vi "Chessy_Drive_Main.vi"(0 "Speed_Main":dbl, 1 "Turning_Main":dbl, 5 "Speed_Limit":dbl, 7 "Turning_Limit":dbl, 12 "Quick_Turn":bool) -> (3 "Left_Motor":dbl format="%.2f", 14 "Right_Motor":dbl format="%.2f")   [LabVIEW 2014]
uses:
  General_VI/Global Var.vi
panel:
  out "Yaw 2":dbl(graph)
  in  "Tune_PID":bool
  out "Yaw":dbl(graph)
  in  "PID Turnin Gains":T1={"proportional gain (Kc)"=0.02, "integral time (Ti, min)"=0.0, "derivative time (Td, min)"=0.003} {"derivative time (Td, min)" format="%.3f"; "integral time (Ti, min)" format="%.3f"; "proportional gain (Kc)" format="%.3f"}
  out "XY Turning":cluster{"Turning X ":dbl[], "Turning Y":dbl[]}(graph)
  out "XY Speed":cluster{"Speed X":dbl[], "Speed Y":dbl[]}(graph)
  in  "Turning Scale":dbl=1.5
  in  "Turning Y":dbl[](array[numeric])=[-0.5, -0.3, -0.1, 0.0, 0.0, 0.0, 0.1, 0.3, 0.5]
  in  "Turning X":dbl[](array[numeric])=[-1.0, -0.75, -0.12, -0.1, 0.0, 0.1, 0.12, 0.75, 1.0]
  in  "Speed Y":dbl[](array[numeric])=[-0.6, -0.4, -0.15, 0.0, 0.0, 0.0, 0.15, 0.4, 0.6]
  in  "Speed X":dbl[](array[numeric])=[-1.0, -0.75, -0.06, -0.05, 0.0, 0.05, 0.06, 0.75, 1.0]
  in  "Turning_Hyd_Deadband":dbl=0.75
  in  "Speed_Hyd_Deadband":dbl=0.75
  out "Delta":dbl format="%.2f"
  # "Chessy Drive"
  # "This subystem takes turning and speed controls from a xbox joystick \nand creats left and right motor values"
  # "Tunning"
  # "Inputs"
  # "Test Points"
  # "Ouputs"
  # "Joystick Map (Lookup Table)"
  # "Hyp Cmd Deadband"
  # "Turning Power Mode"
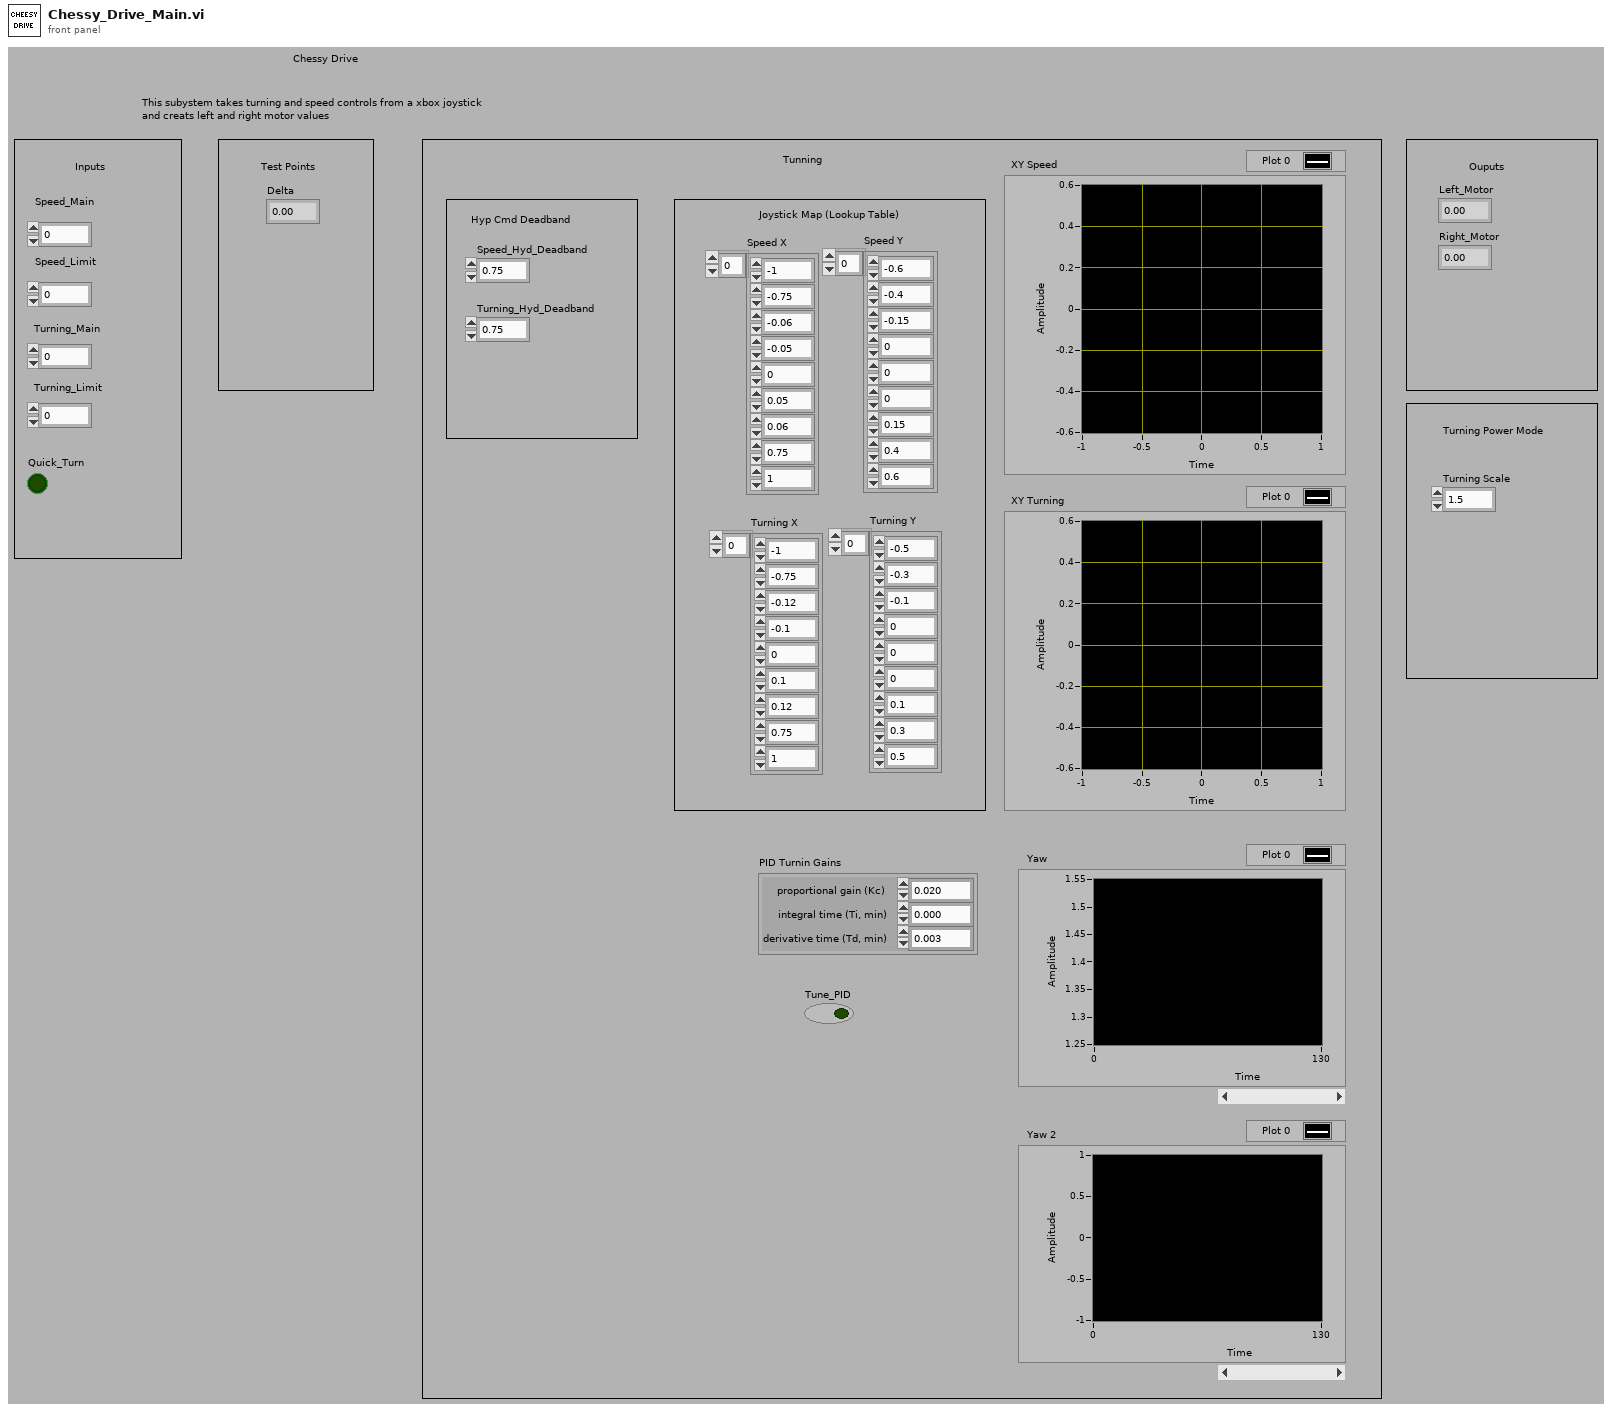
[diagram p1: front panel]
types:
  T1 = cluster{"proportional gain (Kc)":dbl, "integral time (Ti, min)":dbl, "derivative time (Td, min)":dbl}
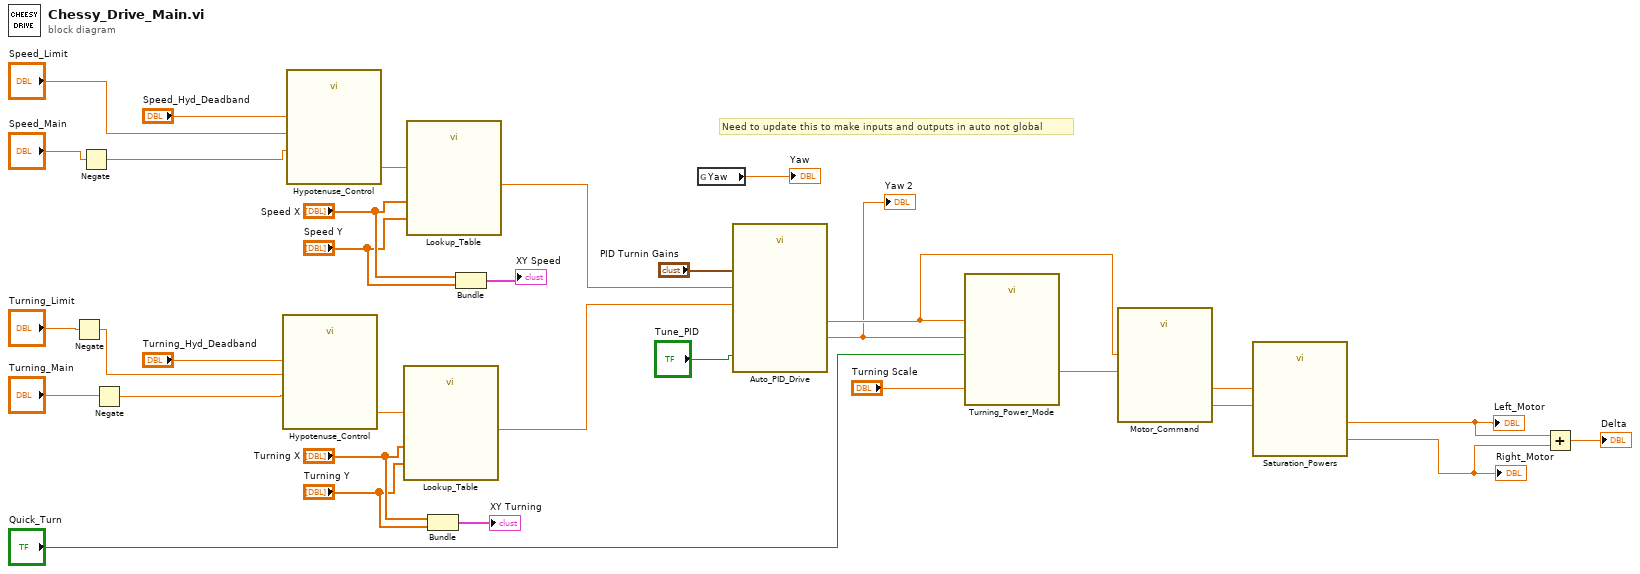
[diagram p0: block diagram]
diagram:
  # "Need to update this to make inputs and outputs in auto not global"
  n1 = Negate(x="Turning_Limit") -> (-x=w16:dbl)
  n2 = Negate(x="Speed_Main") -> (-x=w8:dbl)
  n3 = Negate(x="Turning_Main") -> (-x=w18:dbl)
  n4 = call "Hypotenuse_Control.vi"("Deadband"="Turning_Hyd_Deadband", "Limit_Axis"=w16, "Main_Axis"=w18) -> ("Axis_Adj"=w21:dbl)  [unwired: 8 in]
  n5 = call "Hypotenuse_Control.vi"("Deadband"="Speed_Hyd_Deadband", "Limit_Axis"="Speed_Limit", "Main_Axis"=w8) -> ("Axis_Adj"=w24:dbl)  [unwired: 8 in]
  n6 = call "Lookup_Table.vi"("Y_Array"="Turning Y", "x_in"=w21, "X_Array"="Turning X") -> ("y_out"=w6:dbl)  [unwired: 6 in]
  n7 = call "Lookup_Table.vi"("Y_Array"="Speed Y", "x_in"=w24, "X_Array"="Speed X") -> ("y_out"=w7:dbl)  [unwired: 6 in]
  n8 = Bundle("Turning X"="Turning X", "Turning Y"="Turning Y") -> (→"XY Turning":cluster{"Turning X ":dbl[], "Turning Y":dbl[]})  [unwired: 1 in]
  n9 = Bundle("Speed X"="Speed X", "Speed Y"="Speed Y") -> (→"XY Speed":cluster{"Speed X":dbl[], "Speed Y":dbl[]})  [unwired: 1 in]
  n10 = global read "Global Var.vi" "Yaw"() -> (→"Yaw":dbl)
  n11 = call "Auto_PID_Drive.vi"("Tune_PID"="Tune_PID", "PID Turnin Gains"="PID Turnin Gains", "Turning"=w6, "Power"=w7) -> ("Turning"=w1:dbl, "Power"=w4:dbl)  [unwired: 6 in]
  "Yaw 2" <- w1
  n12 = call "Turning_Power_Mode.vi"("Turning_Scale"="Turning Scale", "Quick_Turn"="Quick_Turn", "Turning"=w1, "Power"=w4) -> ("Turning_Correction"=w28:dbl)  [unwired: 7 in]
  n13 = call "Motor_Command.vi"("Turning"=w28, "Power"=w4) -> ("Right_Motor"=w31:dbl, "Left_Motor"=w29:dbl)  [unwired: 8 in]
  n14 = call "Saturation_Powers.vi"("Right_Motor"=w31, "Left_Motor"=w29) -> ("Right_Motor_Say"=w26:dbl, "Left_Motor_Sat"=w27:dbl)  [unwired: 8 in]
  "Left_Motor" <- w27
  "Right_Motor" <- w26
  n15 = Add(x=w27, y=w26) -> (x+y=→"Delta":dbl)
